vi "GetFloatValue.vi"(0 "nInputHandle":u64, 7 "strName":string, 11 "error in (no error)":errorcluster) -> (4 "nOutputHandle":u64, 6 "dCurValue":dbl, 8 "pstFloatValue":T1, 10 "GX_STATUS":i32, 15 "error out":errorcluster)   [LabVIEW 2016, in "GxLVLib.lvlib"]
uses:
  GxLVLib.lvlib
  GxIAPI.dll
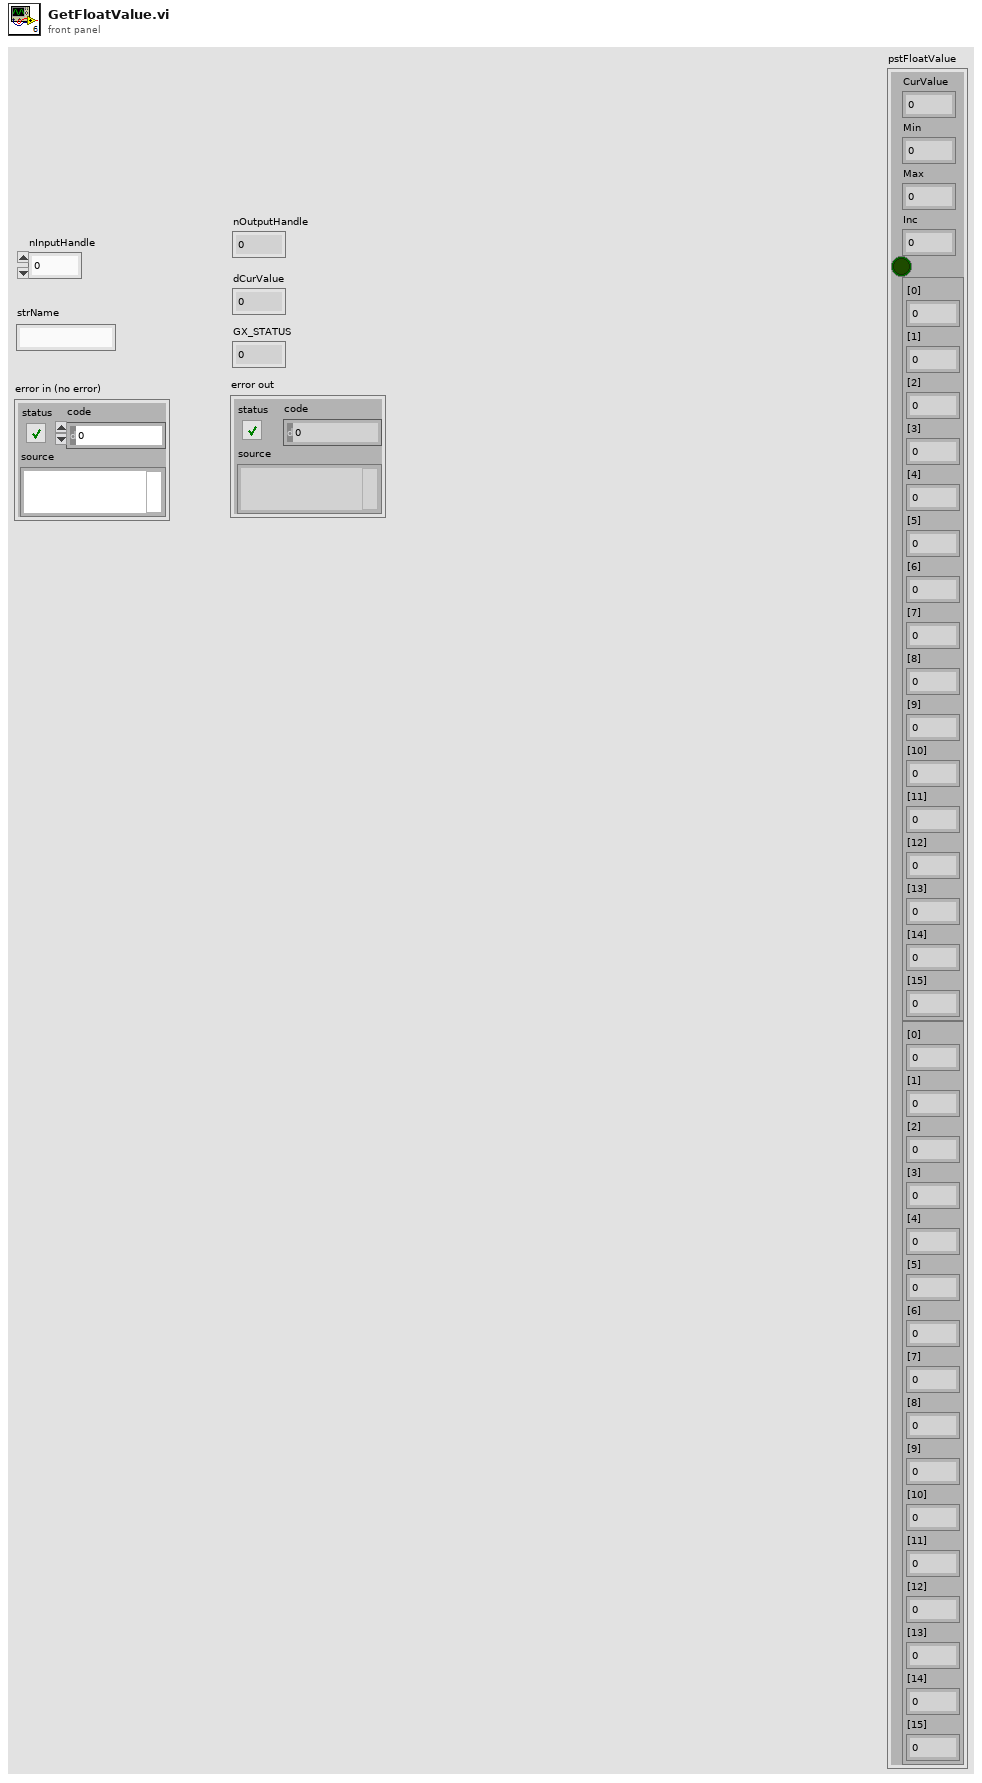
[diagram p1: front panel]
types:
  T1 = cluster{"CurValue":dbl, "Min":dbl, "Max":dbl, "Inc":dbl, bool, cluster{"[0]":i8, "[1]":i8, "[2]":i8, "[3]":i8, "[4]":i8, "[5]":i8, "[6]":i8, "[7]":i8, "[8]":i8, "[9]":i8, "[10]":i8, "[11]":i8, "[12]":i8, "[13]":i8, "[14]":i8, "[15]":i8}, cluster{"[0]":i32, "[1]":i32, "[2]":i32, "[3]":i32, "[4]":i32, "[5]":i32, "[6]":i32, "[7]":i32, "[8]":i32, "[9]":i32, "[10]":i32, "[11]":i32, "[12]":i32, "[13]":i32, "[14]":i32, "[15]":i32}}
  T2 = cluster{"[0]":i8, "[1]":i8, "[2]":i8, "[3]":i8, "[4]":i8, "[5]":i8, "[6]":i8, "[7]":i8, "[8]":i8, "[9]":i8, "[10]":i8, "[11]":i8, "[12]":i8, "[13]":i8, "[14]":i8, "[15]":i8}
  T3 = cluster{"[0]":i32, "[1]":i32, "[2]":i32, "[3]":i32, "[4]":i32, "[5]":i32, "[6]":i32, "[7]":i32, "[8]":i32, "[9]":i32, "[10]":i32, "[11]":i32, "[12]":i32, "[13]":i32, "[14]":i32, "[15]":i32}
  T4 = cluster{"dCurValue":dbl, "dMin":dbl, "dMax":dbl, "dInc":dbl, bool, cluster{"[0]":i8, "[1]":i8, "[2]":i8, "[3]":i8, "[4]":i8, "[5]":i8, "[6]":i8, "[7]":i8, "[8]":i8, "[9]":i8, "[10]":i8, "[11]":i8, "[12]":i8, "[13]":i8, "[14]":i8, "[15]":i8}, cluster{"[0]":i32, "[1]":i32, "[2]":i32, "[3]":i32, "[4]":i32, "[5]":i32, "[6]":i32, "[7]":i32, "[8]":i32, "[9]":i32, "[10]":i32, "[11]":i32, "[12]":i32, "[13]":i32, "[14]":i32, "[15]":i32}}
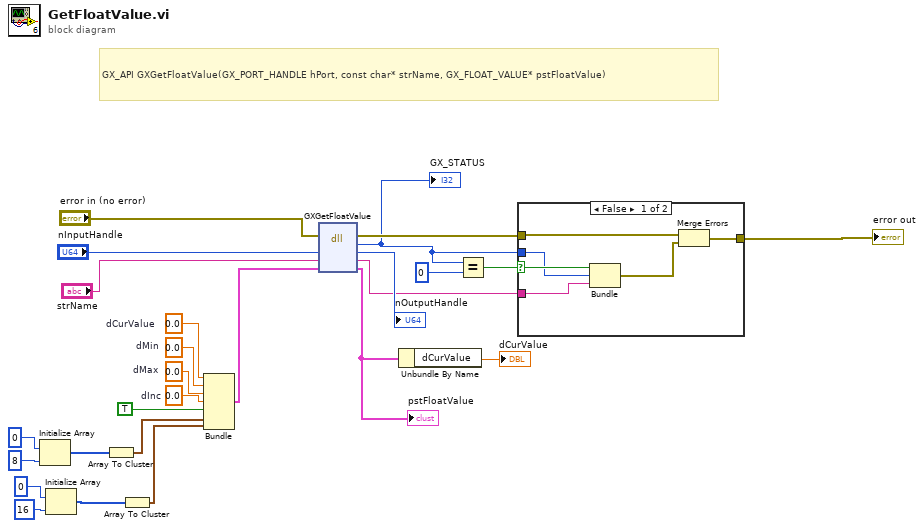
[diagram p0: block diagram]
diagram:
  w23 = 0.0  # dInc
  w24 = 0.0  # dMax
  w25 = 0.0  # dMin
  w26 = 0.0  # dCurValue
  # "GX_API GXGetFloatValue(GX_PORT_HANDLE hPort, const char* strName, GX_FLOAT_VALUE* pstFloatValue)"
  n1 = Initialize Array(i8 0, 8) -> (w8:i8[])
  n2 = Initialize Array(0, 16) -> (w10:i32[])
  n3 = Array To Cluster(array=w8) -> (cluster=w9:T2)
  n4 = Array To Cluster(array=w10) -> (cluster=w11:T3)
  n5 = Bundle("dCurValue"=w26, "dMin"=w25, "dMax"=w24, "dInc"=w23, TRUE, w9, w11) -> (w20:T4)  [unwired: 1 in]
  n6 = dll-call lib="GxIAPI.dll" fn="GXGetFloatValue"(error in="error in (no error)", "hDevice"="nInputHandle", "strName"="strName", "pstFloatValue"=w20) -> (error out=w15:errorcluster, "GX_STATUS"=w4:i32, "hDevice"=→"nOutputHandle":i64, "strName"=w12:string, "pstFloatValue"=w7:T4)  [unwired: 2 in, 1 out]
  "GX_STATUS" <- w4
  "pstFloatValue" <- w7
  n7 = Unbundle By Name(w7) -> ("dCurValue"=→"dCurValue":dbl)
  n8 = Equal?(x=w4, y=0) -> (x = y?=w13:bool)
  n9 = case shown="False" w13 {
    selector: w13 -> [w29 _]
    tunnel: w15 -> [w32 w33]
    tunnel: [w31 w33] -> w5
    tunnel: w4 -> [w28 _]
    tunnel: w12 -> [w27 _]
    frame False {
      n10 = Bundle(w29, "GX_STATUS"=w28, "strName"=w27) -> (w30:cluster{bool, "GX_STATUS":i32, "strName":string})  [unwired: 1 in]
      n11 = Merge Errors(w32, w30) -> (w31:errorcluster)
    }
    frame True {
    }
  }
  "error out" <- w5
